vi "Publish Method Result.vi"(10 "Test Method Result":T1, 11 "Slave Test Runner In":refnum<class "Slave Test Runner.lvclass">) -> (3 "Slave Test Runner Out":refnum<class "Slave Test Runner.lvclass">)   [LabVIEW 2020, in "Slave Test Runner.lvclass"]
uses:
  Slave Test Runner.lvclass
  Result Types/Method Result/Method Result.ctl
  Result Types/Assertion Result/Public/TypeDefs/Status.ctl
  Result Types/Assertion Result/Assertion Result.ctl
  Result Types/Assertion Result/Public/TypeDefs/Assertion Type.ctl
  Slave Test Runner.lvclass/Slave Test Runner.ctl
  Result Collector/Result Collector.lvclass/Result Collector.ctl
  Result Collector/Result Collector.lvclass
  Result Types/Assertion Result/Assertion Result.lvlib
  Result Types/Method Result/Method Result.lvlib
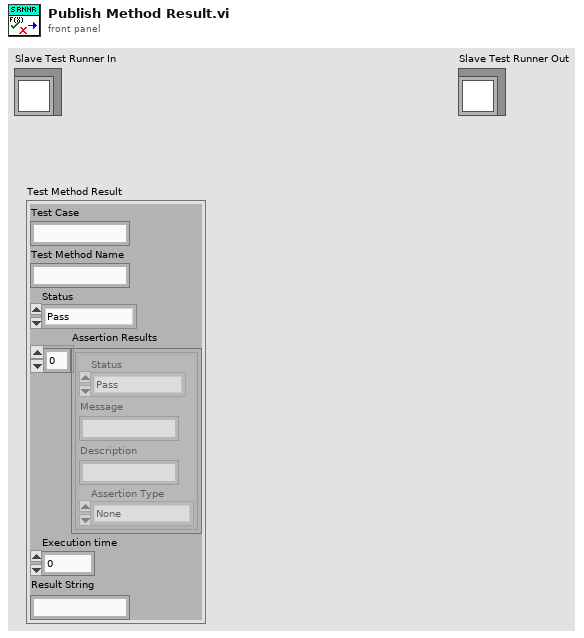
[diagram p1: front panel]
types:
  T1 = typedef "Method Result.lvlib/Method Result.ctl" = cluster{"Test Case":string, "Test Method Name":string, "Status":T2, "Assertion Results":T3[], "Execution time":dbl, "Result String":string}
  T2 = typedef "Assertion Result.lvlib/Status.ctl" = enum16{"Pass", "Fail", "Error", "Skipped", "Setup Error", "Broken", "Teardown Error"}
  T3 = typedef "Assertion Result.lvlib/Assertion Result.ctl" = cluster{"Status":T2, "Message":string, "Description":string, "Assertion Type":T4}
  T4 = typedef "Assertion Result.lvlib/Assertion Type.ctl" = enum16{"None", "Pass", "Fail", "Skip", "Pass if Equal", "Fail if Equal", "Pass if Error", "Fail if Error", "Pass if", "Fail if"}
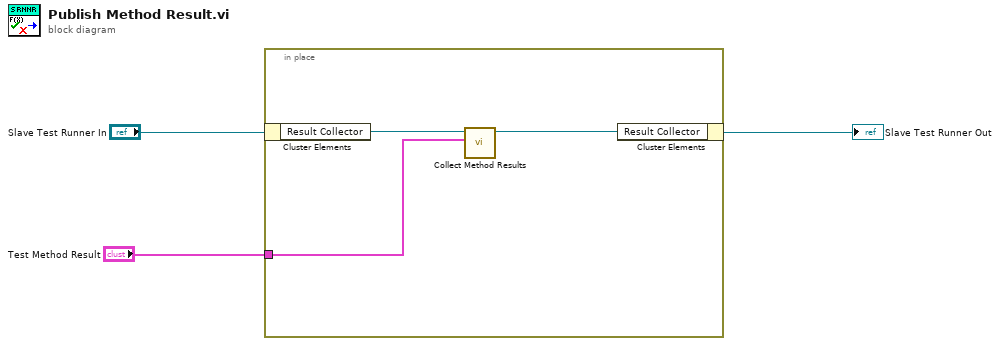
[diagram p0: block diagram]
diagram:
  n1 = in-place {
    in-place-border: "Test Method Result" -> [w4]
    n2 = in-place-cluster #1("Slave Test Runner In") -> ("Result Collector"=w6:refnum<class "Result Collector.lvclass">)
    n3 = call "Collect Method Results.vi"("Test Method Result"=w4, "Report Generator In"=w6) -> ("Report Generator Out"=w5:refnum<class "Result Collector.lvclass">)  [unwired: 9 in]
    n4 = in-place-cluster #1("Result Collector"=w5) -> (→"Slave Test Runner Out":refnum<class "Slave Test Runner.lvclass">)
  }
